vi "Release Lock.vi"(8 "error in (no error)":errorcluster, 9 "timeout (0 ms)":i32 format="%d ms", 10 "new lock status (T)":bool=TRUE, 11 "Pointer in":refnum<class "Pointer.lvclass">) -> (0 "error out":errorcluster, 1 "timed out?":bool, 3 "Pointer out":refnum<class "Pointer.lvclass">)   [LabVIEW 2017, in "Memory Manager.lvlib" / "Pointer.lvclass"]
uses:
  Pointer.lvclass
  Pointer.lvclass/Pointer.ctl
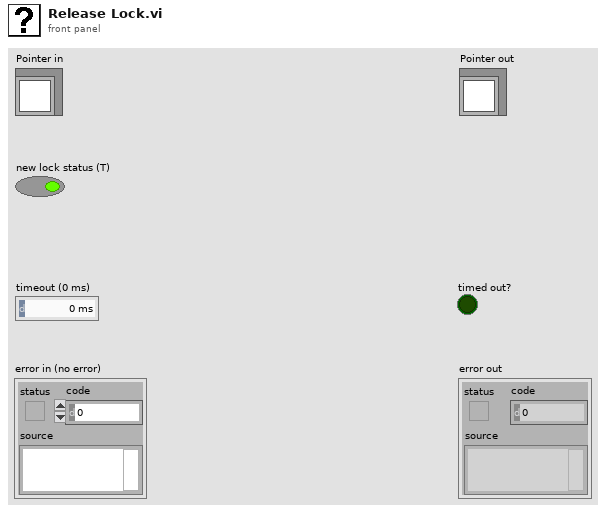
[diagram p1: front panel]
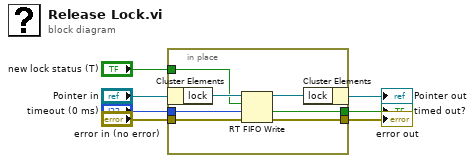
[diagram p0: block diagram]
diagram:
  n1 = in-place {
    in-place-border: "error in (no error)" -> [w14]
    in-place-border: [w10] -> w3
    in-place-border: "timeout (0 ms)" -> [w13]
    in-place-border: [w9] -> w2
    in-place-border: "new lock status (T)" -> [w8]
    n2 = in-place-cluster #1("Pointer in") -> ("lock"=w12:refnum<k33>)
    n3 = RT FIFO Write(0:w12, 1:w8, 2:w13, 3:w14) -> (8:w11:refnum<k33>, 10:w9:bool, 11:w10:errorcluster)  [unwired: 1 in, 1 out]
    n4 = in-place-cluster #1("lock"=w11) -> (→"Pointer out":refnum<class "Pointer.lvclass">)
  }
  "error out" <- w3
  "timed out?" <- w2
